vi "RTM FramePopUp.vi"(8 "error in (no error)":errorcluster, 9 "NETWORK --> DUT Frames":T2[](array[typedef]), 10 "DUT --> NETWORK Frames":T2[](array[typedef]), 11 "Node Ptr":T1 format="%.0x") -> (0 "error out":errorcluster, 3 "Node Ptr 2":T1 format="%.0x")   [LabVIEW 2018, in "CAN Gateway System Explorer.lvlib"]
uses:
  CAN Gateway System Explorer.lvlib
  Types/FramesCluster.ctl
  <vilib>/NI Veristand/Custom Device API/Custom Device Item Ref.ctl
  Types/Frame Controls.ctl
  Shared/Constants.vi
  <vilib>/NI Veristand/Custom Device API/Get Item Property (Variant).vi
  <vilib>/NI Veristand/Custom Device API/Get Item Property (String).vi
  <vilib>/NI Veristand/Custom Device API/Set Item Property (Variant).vi
  <vilib>/NI Veristand/Custom Device API/Custom Device API.lvlib
  Shared/CAN Gateway Shared.lvlib
panel:
  in  "Cancel Button":bool
  in  "OK Button":bool
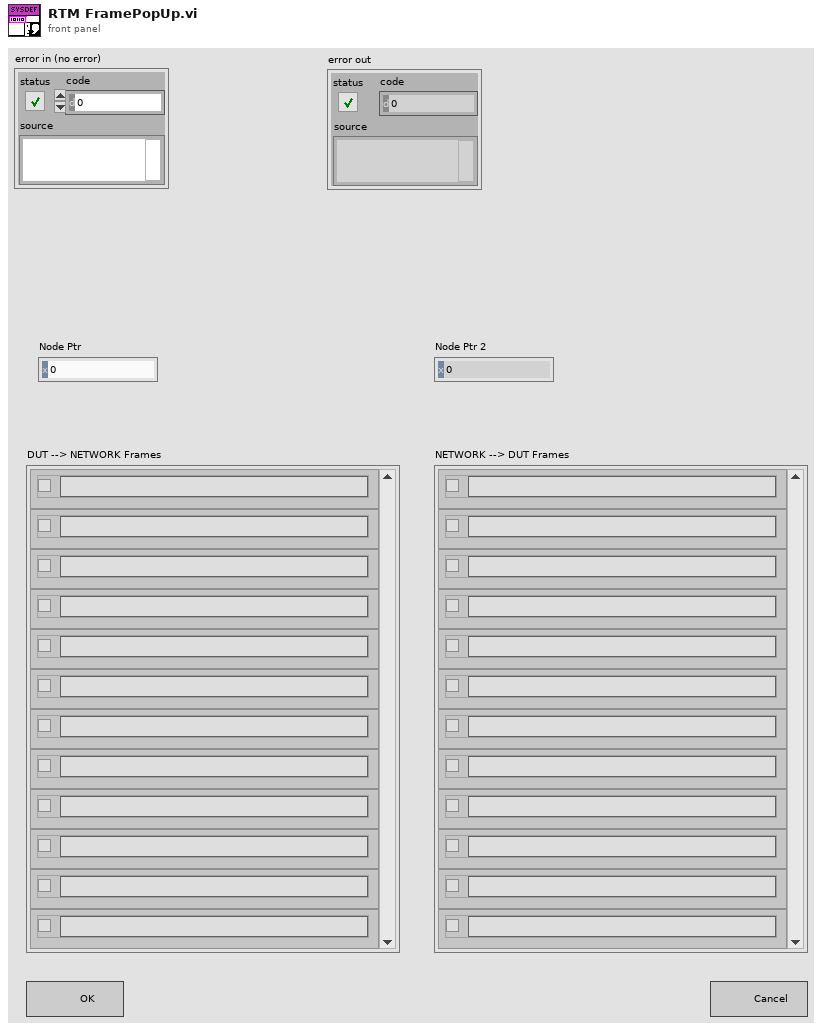
[diagram p1: front panel]
types:
  T1 = typedef "Custom Device API.lvlib/Custom Device Item Ref.ctl" = u64
  T2 = typedef "CAN Gateway System Explorer.lvlib/FramesCluster.ctl" = cluster{"Frame":string, "Fault":bool}
  T3 = typedef "CAN Gateway System Explorer.lvlib/Frame Controls.ctl" = refnum<vi>[]
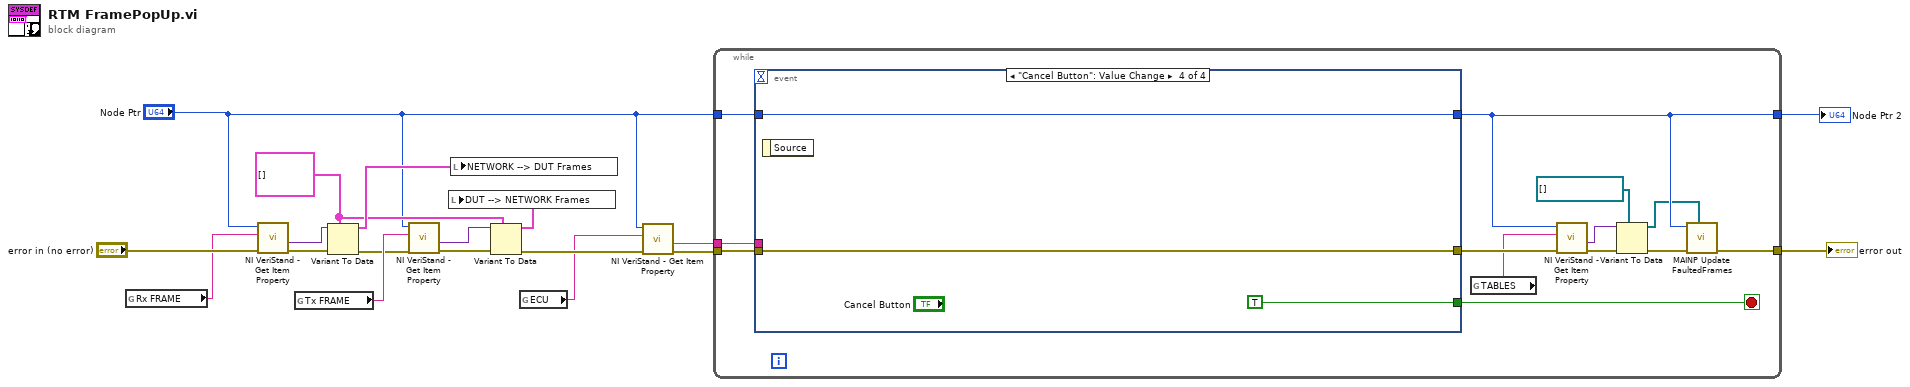
[diagram p0: block diagram]
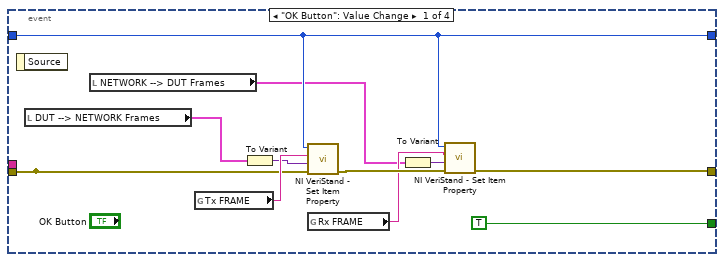
[diagram p2: hidden frame]
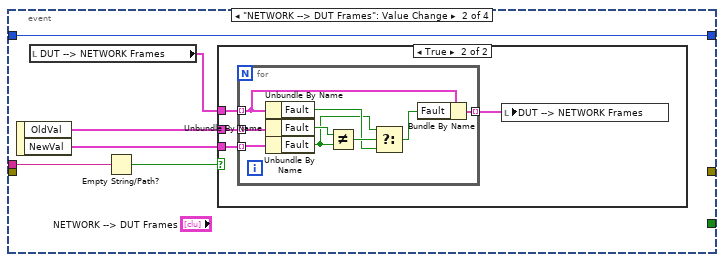
[diagram p3: hidden frame]
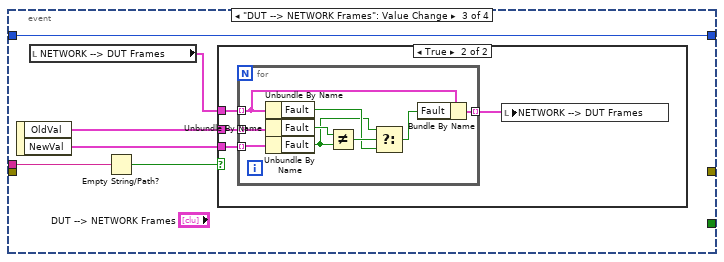
[diagram p5: hidden frame]
diagram:
  w8 = T2[] []
  n1 = global read "Constants.vi" "Rx FRAME"() -> (w11:string)
  n2 = call-poly <vilib>:"NI VeriStand - Get Item Property.vi"("error in (no error)"="error in (no error)", "Property Name"=w11, "Item Ref in"="Node Ptr") -> ("error out"=w13:errorcluster, "Value"=w14:variant)  [unwired: 5 in, 2 out]
  n3 = global read "Constants.vi" "Tx FRAME"() -> (w17:string)
  n4 = Variant To Data(error in=w13, type=w8, Variant=w14) -> (data=w10:T2[], error out=w15:errorcluster)
  n5 = call-poly <vilib>:"NI VeriStand - Get Item Property.vi"("error in (no error)"=w15, "Property Name"=w17, "Item Ref in"="Node Ptr") -> ("error out"=w16:errorcluster, "Value"=w18:variant)  [unwired: 5 in, 2 out]
  n6 = local write "NETWORK --> DUT Frames"(w10) -> ()
  n7 = Variant To Data(error in=w16, type=w8, Variant=w18) -> (data=w9:T2[], error out=w5:errorcluster)
  n8 = local write "DUT --> NETWORK Frames"(w9) -> ()
  n9 = global read "Constants.vi" "ECU"() -> (w3:string)
  n10 = call-poly <vilib>:"NI VeriStand - Get Item Property.vi"("error in (no error)"=w5, "Property Name"=w3, "Item Ref in"="Node Ptr") -> ("error out"=w4:errorcluster, "Value"=w1:string)  [unwired: 5 in, 2 out]
  n11 = while {
    tunnel: w4 -> [w30]
    tunnel: "Node Ptr" -> [w29]
    tunnel: [w25] -> w6
    tunnel: [w26] -> w7
    tunnel: w1 -> [w19]
    stop <- w31 stop-if-true
    n12 = event shown="[3] \"Cancel Button\": Value Change" {
      selector: _ -> [_ _ _ _]
      dyn-events: _ -> [_ _ _ _]
      timeout: _ -> [_ _ _ _]
      tunnel: [w34 _ _ w82] -> w28
      tunnel: [TRUE _ _ TRUE] -> w31
      tunnel: w30 -> [w39 _ _ w82]
      tunnel: w29 -> [w36 w45 w64 w81]
      tunnel: [w36 w45 w64 w81] -> w25
      tunnel: [w39 _ _ _] -> _
      tunnel: w19 -> [_ w47 w66 _]
      event "OK Button": Value Change {
        n13 = event-data() -> ()  [unwired: 1 in, 1 out]
        n14 = local read "DUT --> NETWORK Frames"() -> (w32:T2[])
        n15 = local read "NETWORK --> DUT Frames"() -> (w33:T2[])
        n16 = global read "Constants.vi" "Tx FRAME"() -> (w41:string)
        n17 = To Variant(anything=w32) -> (Variant=w40:variant)
        n18 = call-poly <vilib>:"NI VeriStand - Set Item Property.vi"("error in (no error)"=w39, "Value"=w40, "Property Name"=w41, "Item Ref in"=w36) -> ("error out"=w37:errorcluster)  [unwired: 5 in, 2 out]
        n19 = global read "Constants.vi" "Rx FRAME"() -> (w35:string)
        n20 = To Variant(anything=w33) -> (Variant=w38:variant)
        n21 = call-poly <vilib>:"NI VeriStand - Set Item Property.vi"("error in (no error)"=w37, "Value"=w38, "Property Name"=w35, "Item Ref in"=w36) -> ("error out"=w34:errorcluster)  [unwired: 5 in, 2 out]
      }
      event "NETWORK --> DUT Frames": Value Change {
        n22 = event-data() -> ("OldVal"=w48:T2[], "NewVal"=w44:T2[])  [unwired: 1 in]
        n23 = local read "DUT --> NETWORK Frames"() -> (w43:T2[])
        n24 = Empty String/Path?(string/path=w47) -> (empty?=w46:bool)
        n25 = case shown="True" w46 {
          tunnel: w48 -> [_ w52]
          tunnel: w44 -> [_ w51]
          tunnel: w43 -> [_ w50]
          frame False {
          }
          frame True {
            n26 = for {
              tunnel: w52 -> [w60] mode=indexing
              tunnel: w51 -> [w61] mode=indexing
              tunnel: w50 -> [w57] mode=indexing
              tunnel: [w55] -> w49 mode=indexing
              n27 = Unbundle By Name(w57) -> ("Fault"=w58:bool)
              n28 = Unbundle By Name(w60) -> ("Fault"=w54:bool)
              n29 = Unbundle By Name(w61) -> ("Fault"=w53:bool)
              n30 = Not Equal?(x=w54, y=w53) -> (x != y?=w59:bool)
              n31 = Select(t=w53, s=w59, f=w58) -> (s? t:f=w56:bool)
              n32 = Bundle By Name(cluster=w57, "Fault"=w56) -> (w55:T2)
            }
            n33 = local write "DUT --> NETWORK Frames"(w49) -> ()
          }
        }
      }
      event "DUT --> NETWORK Frames": Value Change {
        n34 = event-data() -> ("OldVal"=w67:T2[], "NewVal"=w63:T2[])  [unwired: 1 in]
        n35 = local read "NETWORK --> DUT Frames"() -> (w62:T2[])
        n36 = Empty String/Path?(string/path=w66) -> (empty?=w65:bool)
        n37 = case shown="True" w65 {
          tunnel: w67 -> [_ w71]
          tunnel: w63 -> [_ w70]
          tunnel: w62 -> [_ w69]
          frame False {
          }
          frame True {
            n38 = for {
              tunnel: w71 -> [w79] mode=indexing
              tunnel: w70 -> [w80] mode=indexing
              tunnel: w69 -> [w76] mode=indexing
              tunnel: [w74] -> w68 mode=indexing
              n39 = Unbundle By Name(w76) -> ("Fault"=w77:bool)
              n40 = Unbundle By Name(w79) -> ("Fault"=w73:bool)
              n41 = Unbundle By Name(w80) -> ("Fault"=w72:bool)
              n42 = Not Equal?(x=w73, y=w72) -> (x != y?=w78:bool)
              n43 = Select(t=w72, s=w78, f=w77) -> (s? t:f=w75:bool)
              n44 = Bundle By Name(cluster=w76, "Fault"=w75) -> (w74:T2)
            }
            n45 = local write "NETWORK --> DUT Frames"(w68) -> ()
          }
        }
      }
      event "Cancel Button": Value Change {
        n46 = event-data() -> ()  [unwired: 1 in, 1 out]
      }
    }
    n47 = global read "Constants.vi" "TABLES"() -> (w27:string)
    n48 = call-poly <vilib>:"NI VeriStand - Get Item Property.vi"("error in (no error)"=w28, "Property Name"=w27, "Item Ref in"=w25) -> ("error out"=w24:errorcluster, "Value"=w22:variant)  [unwired: 5 in, 2 out]
    n49 = Variant To Data(error in=w24, type=T3 [] ("Array"), Variant=w22) -> (data=w20:T3, error out=w23:errorcluster)
    n50 = call "MAINP Update FaultedFrames.vi"("Controls"=w20, "error in (no error)"=w23, "Device Item Ref in"=w25) -> ("error out"=w26:errorcluster)  [unwired: 7 in, 1 out]
  }
  "error out" <- w7
  "Node Ptr 2" <- w6
